vi "Build SPI Configuration.vi"(8 "error in (no error)":errorcluster, 11 "Item Ref in":T1 format="%.0x") -> (0 "error out":errorcluster, 2 "SPI Configuration":refnum<k24>, 3 "Item Ref out":T1 format="%.0x")   [LabVIEW 2014, in "SLSC configuration System Explorer.lvlib"]
uses:
  SLSC configuration System Explorer.lvlib
  <vilib>/NI Veristand/Custom Device API/Custom Device Item Ref.ctl
  <vilib>/NI Veristand/Custom Device API/Custom Device API.lvlib
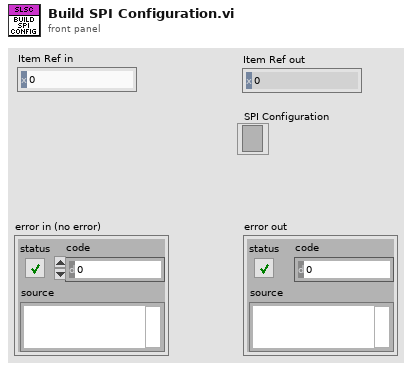
[diagram p1: front panel]
types:
  T1 = typedef "Custom Device API.lvlib/Custom Device Item Ref.ctl" = u64
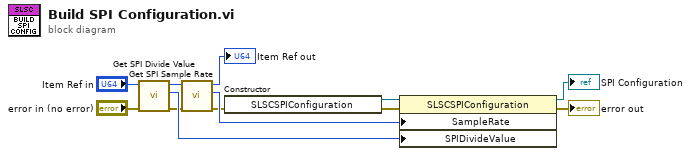
[diagram p0: block diagram]
diagram:
  n1 = call "Get SPI Divide Value.vi"("error in (no error)"="error in (no error)", "Device Ref in"="Item Ref in") -> ("error out"=w8:errorcluster, "SPI Divide Value"=w11:u16, "Item Ref out"=w9:T1)  [unwired: 7 in]
  n2 = call "Get SPI Sample Rate.vi"("error in (no error)"=w8, "Item Ref in"=w9) -> ("error out"=w10:errorcluster, "SPI Sample Rate"=w12:u32, "Item Ref out"=→"Item Ref out":T1)  [unwired: 7 in]
  n3 = constructor class="SLSCSPIConfiguration"(error in=w10) -> (reference out=w5:refnum<k24>, error out=w4:errorcluster)  [unwired: 2 in, 1 out]
  n4 = property class="SLSCSPIConfiguration"(reference=w5, error in=w4, "SampleRate"=w12, "SPIDivideValue"=w11) -> (reference out=→"SPI Configuration":refnum<k24>, error out=→"error out":errorcluster)
